vi "Agilent 33XXX Series Generate Frequency Sweep - SW Triggered.vi"() -> ()   [LabVIEW 2020, in "AWG.lvlib"]
doc: "Shows how to configure and enable a triggered frequency sweep.\n\nNote:\n\nOutput is always enabled on model 33120, so the standard waveform will appear for a short amount of time before the first trigger is received for the frequency sweep."
uses:
  AWG.lvlib
  Agilent 33XXX Series.lvlib
panel:
  in  "Serial Configuration":T1={"Baud Rate"=9600, "Parity"=0, "Data Bits"=8, "Flow Control"=4} {"Flow Control" items=["None", "XON/XOFF", "RTS/CTS", "XON/XOFF & RTS/CTS", "DTR/DSR", "XON/XOFF & DTR/DSR"]; "Data Bits" items=["7"=7, "8"=8]; "Parity" items=["None", "Odd", "Even", "Mark", "Space"]; "Baud Rate" items=["300"=300, "600"=600, "1200"=1200, "2400"=2400, "4800"=4800, "9600"=9600, "19200"=19200]}
  in  "Waveform Function (1: Sine)":u16(ring)=1 items=["DC", "Sine", "Square", "Triangle", "Ramp", "Pulse", "Noise", "Sinc", "Negative Ramp", "Exponential Rise", "Exponential Fall", "Cardiac"]
  in  "Stop  Frequency  (1000.0 Hz)":dbl=1000.0 format="%#.6g"
  in  "Start Frequency (100.0 Hz)":dbl=100.0 format="%#.6g"
  in  "Sweep Time (1.00 s)":dbl=1.0 format="%#.6g"
  in  "Amplitude (1 Vpp)":dbl=1.0
  in  "VISA resource name":refnum<visa-resource-name>
  # "(c) 2005 - 2013 National Instruments.  ALL RIGHTS RESERVED."
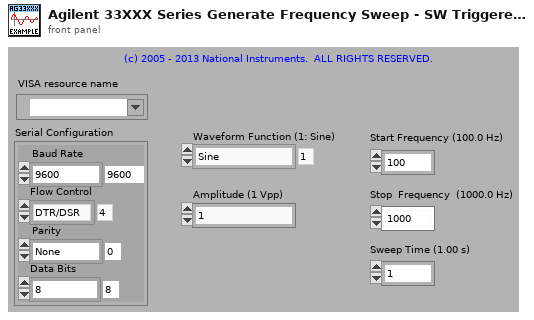
[diagram p1: front panel]
types:
  T1 = cluster{"Baud Rate":u32, "Parity":u16, "Data Bits":u16, "Flow Control":u16}
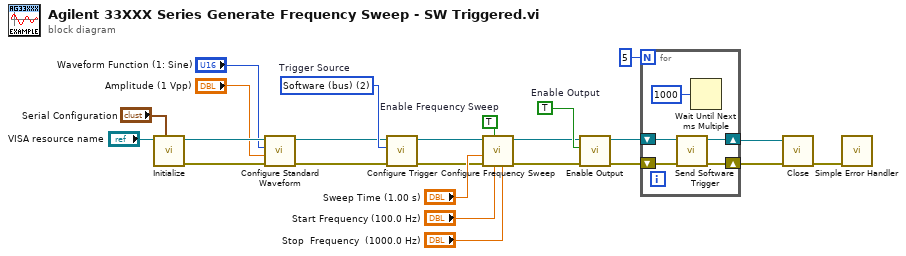
[diagram p0: block diagram]
diagram:
  w8 = TRUE  # Enable Output
  w17 = u16 2 items=["Internal", "External", "Software (bus)"]  # Trigger Source
  w20 = TRUE  # Enable Frequency Sweep
  n1 = call "Initialize.vi"("Serial Configuration"="Serial Configuration", "VISA resource name"="VISA resource name") -> ("error out"=w21:errorcluster, "VISA resource name out"=w24:refnum<visa-resource-name>)  [unwired: 7 in, 1 out]
  n2 = call "Configure Standard Waveform.vi"("error in (no error)"=w21, "Amplitude (1)"="Amplitude (1 Vpp)", "Waveform Function (1: Sine)"="Waveform Function (1: Sine)", "VISA resource name"=w24) -> ("error out"=w3:errorcluster, "VISA resource name out"=w4:refnum<visa-resource-name>)  [unwired: 6 in]
  n3 = call "Configure Trigger.vi"("error in (no error)"=w3, "Trigger Source (0: Internal)"=w17, "VISA resource name"=w4) -> ("error out"=w1:errorcluster, "VISA resource name out"=w2:refnum<visa-resource-name>)  [unwired: 7 in]
  n4 = call "Configure Frequency Sweep.vi"("Stop  Frequency (1000.0 Hz)"="Stop  Frequency  (1000.0 Hz)", "Start Frequency (100.0 Hz)"="Start Frequency (100.0 Hz)", "Enable Frequency Sweep Mode (T: Enable)"=w20, "error in (no error)"=w1, "Sweep Time (1.00 s)"="Sweep Time (1.00 s)", "VISA resource name"=w2) -> ("error out"=w5:errorcluster, "VISA resource name out"=w6:refnum<visa-resource-name>)  [unwired: 4 in]
  n5 = call "Enable Output.vi"("error in (no error)"=w5, "Enable Output  (T: Enable)"=w8, "VISA resource name"=w6) -> ("error out"=w10:errorcluster, "VISA resource name out"=w19:refnum<visa-resource-name>)  [unwired: 7 in]
  n6 = for {
    N: 5 -> [_]
    shift-right: [w27] -> w16
    shift-left: w10 -> [w25]
    shift-right: [w28] -> w15
    shift-left: w19 -> [w29]
    n7 = call "Send Software Trigger.vi"("error in (no error)"=w25, "VISA resource name"=w29) -> ("error out"=w27:errorcluster, "VISA resource name out"=w28:refnum<visa-resource-name>)  [unwired: 8 in]
    n8 = Wait Until Next ms Multiple(millisecond multiple=u32 1000) -> ()  [unwired: 1 out]
  }
  n9 = call "Close.vi"("error in (no error)"=w16, "VISA resource name"=w15) -> ("error out"=w23:errorcluster)  [unwired: 9 in]
  n10 = call <vilib>:"Simple Error Handler.vi"("error in (no error)"=w23) -> ()  [unwired: 4 in, 5 out]
